vi "Untitled 5.vi"(8 "error in":errorcluster, 11 "Resources in":T1 {"ZI ModHandle"."ModHandle" format="0x%08x"; "ZI ModHandle"."Conn" format="0x%08x"; "ZI Handle"."Handle" format="0x%08x"; "ZI Handle"."Conn" format="0x%08x"}) -> (0 "error out":errorcluster, 2 "ZI Data":T4, 3 "Resources out":T1 {"ZI ModHandle"."ModHandle" format="0x%08x"; "ZI ModHandle"."Conn" format="0x%08x"; "ZI Handle"."Handle" format="0x%08x"; "ZI Handle"."Conn" format="0x%08x"})   [LabVIEW 2021]
uses:
  Main/Ver_1/ZI_Data.ctl
  Main/Ver_1/Resources.ctl
  <instrlib>/Zurich Instruments LabOne/Public/ziTypeHandle.ctl
  <instrlib>/Zurich Instruments LabOne/Public/Modules/ziTypeModHandle.ctl
  <instrlib>/Zurich Instruments LabOne/Public/Modules/ziModGetDoubleData.vi
  <instrlib>/Zurich Instruments LabOne/Public/Utility/ziTicksToS_vector.vi
  <instrlib>/Zurich Instruments LabOne/Zurich Instruments LabOne.lvlib
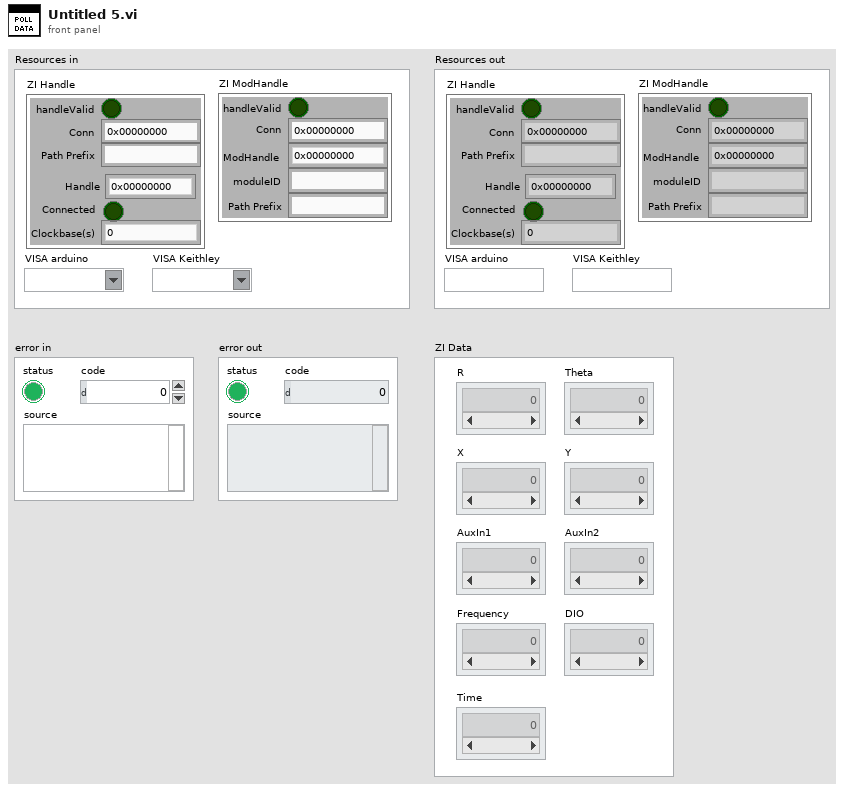
[diagram p1: front panel]
types:
  T1 = typedef "Resources.ctl" = cluster{"ZI Handle":T2, "ZI ModHandle":T3, "VISA arduino":refnum<visa-resource-name>, "VISA Keithley":refnum<visa-resource-name>}
  T2 = typedef "Zurich Instruments LabOne.lvlib/ziTypeHandle.ctl" = cluster{"handleValid":bool, "Conn":u64, "Path Prefix":string, "Handle":u64, "Connected":bool, "Clockbase(s)":dbl}
  T3 = typedef "Zurich Instruments LabOne.lvlib/ziTypeModHandle.ctl" = cluster{"handleValid":bool, "Conn":u64, "ModHandle":u64, "moduleID":string, "Path Prefix":string}
  T4 = typedef "ZI_Data.ctl" = cluster{"R":dbl[], "Theta":dbl[], "X":dbl[], "Y":dbl[], "AuxIn1":dbl[], "AuxIn2":dbl[], "Frequency":dbl[], "DIO":dbl[], "Time":dbl[]}
  T5 = typedef "Zurich Instruments LabOne.lvlib/ziTypeModResults.ctl" = cluster{"PathArray":string[], "ValueType":T6, "NoOfResults":u64, "ziGenericHeader":T7[]}
  T6 = typedef "Zurich Instruments LabOne.lvlib/ziTypePollType.ctl" = enum16{"NONE", "DOUBLE_DATA", "INTEGER_DATA", "DEMOD_SAMPLE", "SCOPE_WAVE_HF2", "AUXIN_SAMPLE", "DIO_SAMPLE", "BYTE_ARRAY", "PWA_WAVE", "9", "10", "11", "12", "13", "14", "15", "TREE_CHANGE_DEPRI", "17", "ERROR", "19", "20", "21", "22", "23", "24", "25", "26", "27", "28", "29", "30", "31", "DOUBLE_DATA_TS", "INTEGER_DATA_TS", "34", "SCOPE_WAVE", "SCOPE_WAVE_EX", "37", "BYTE_ARRAY_TS", "39", "40", "41", "42", "43", "44", "45", "CNT_DATA", "47", "TREE_CHANGE", "49", "50", "51", "52", "53", "54", "55", "56", "57", "58", "59", "60", "61", "62", "63", "SWEEPER_DATA", "SPECTRUM_DATA", "ADVISOR_DATA", "VECTOR_DATA", "IMP_DATA"}
  T7 = typedef "Zurich Instruments LabOne.lvlib/ziTypeModGenericHeader.ctl" = cluster{"HeaderType":enum8{"HEADER_TYPE_NONE", "HEADER_TYPE_SWTRIGGER", "HEADER_TYPE_SWEEPER"}, "SampleFormat":u8, "SystemTime":timestamp, "CreatedTimeStamp":u64, "ChangedTimeStamp":u64, "Flags":u32, "ChunkSizeBytes":u64, "Name":string, "Status":u32, "GroupIndex":u32, "Color":u32, "ActiveRow":u32, "TriggerNumber":u64, "GridRows":u32, "GridCols":u32, "GridMode":u32, "GridOperation":u32, "GridDirection":u32, "GridRepetitions":u32, "GridColDelta":dbl, "GridColOffset":dbl, "GridRowDelta":dbl, "GridRowOffset":dbl, "Bandwidth":dbl, "Center":dbl, "Nenbw":dbl}
  T8 = typedef "Zurich Instruments LabOne.lvlib/ziTypeDoubleDataTS.ctl" = cluster{"Timestamp (ticks)":u64[], "Value":dbl[]}
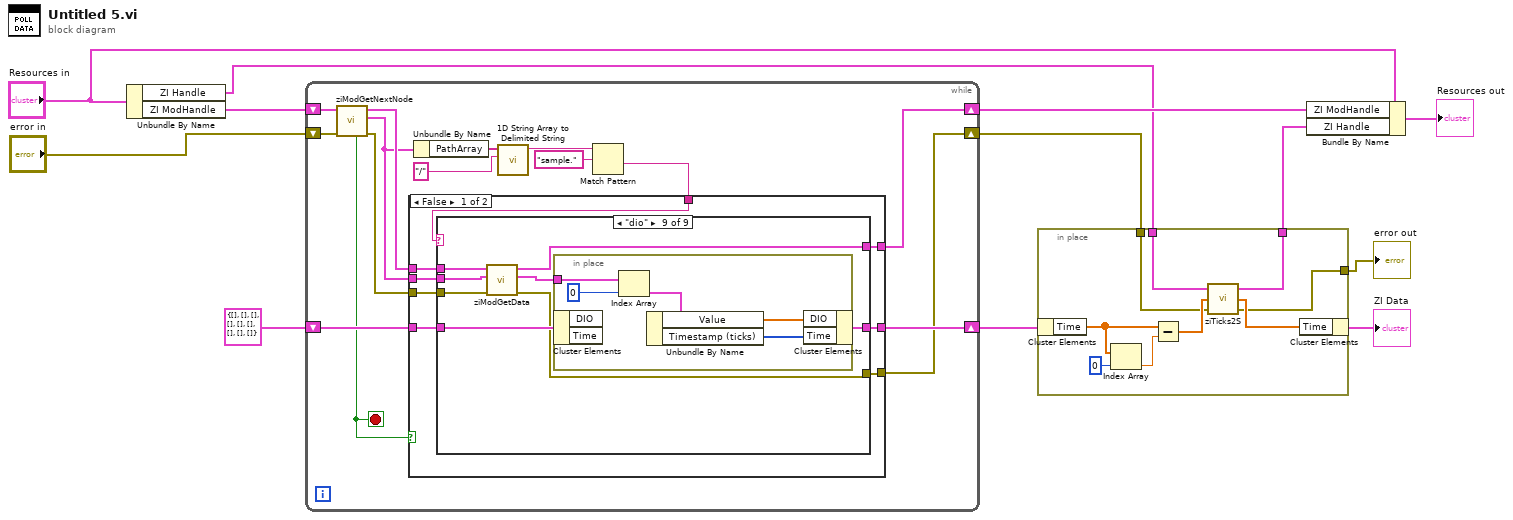
[diagram p0: block diagram]
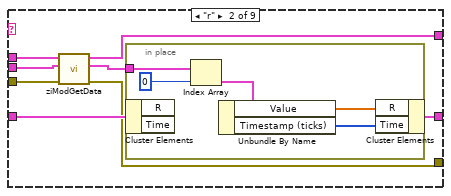
[diagram p3: hidden frame]
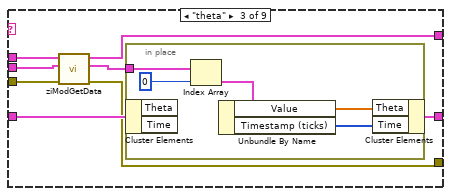
[diagram p4: hidden frame]
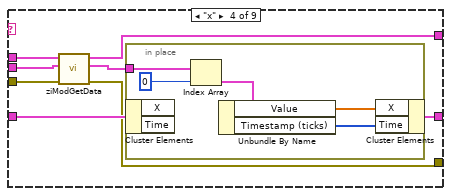
[diagram p5: hidden frame]
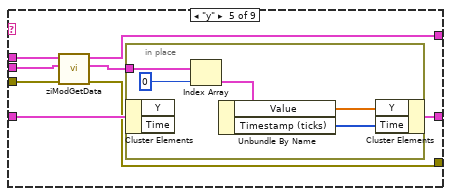
[diagram p6: hidden frame]
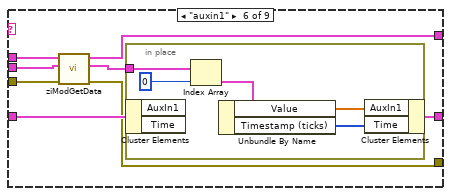
[diagram p7: hidden frame]
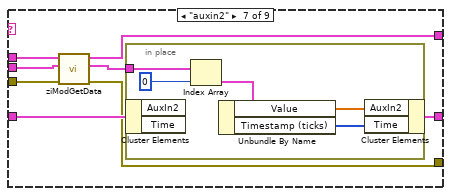
[diagram p8: hidden frame]
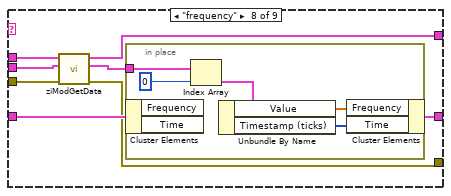
[diagram p9: hidden frame]
diagram:
  n1 = Unbundle By Name("Resources in") -> ("ZI Handle"=w8:T2, "ZI ModHandle"=w12:T3)
  n2 = while {
    shift-right: [w17] -> w10
    shift-left: w12 -> [w27]
    shift-right: [w16] -> w5
    shift-left: "error in" -> [w26]
    shift-right: [w18] -> w9
    shift-left: T4 {"R"=[], "Theta"=[], "X"=[], "Y"=[], "AuxIn1"=[], "AuxIn2"=[], "Frequency"=[], "DIO"=[], "Time"=[]} ("ZI Data") -> [w19]
    stop <- w15 stop-if-true
    n3 = call <instrlib>:"ziModGetNextNode.vi"("Error In"=w26, "ModHandle In"=w27) -> ("Error Out"=w22:errorcluster, "ModResults"=w20:T5, "ModHandle Out"=w21:T3, "NoData"=w15:bool)  [unwired: 6 in]
    n4 = Unbundle By Name(w20) -> ("PathArray"=w23:string[])
    n5 = call <vilib>:"1D String Array to Delimited String.vi"("delimiter"="/", "string array"=w23) -> ("delimited string"=w13:string)  [unwired: 9 in]
    n6 = Match Pattern(string=w13, regular expression="sample.") -> (after substring=w14:string)  [unwired: 1 in, 3 out]
    n7 = case shown="False" w15 {
      tunnel: w14 -> [w35 _]
      tunnel: w22 -> [w33 w144]
      tunnel: w21 -> [w34 w143]
      tunnel: w20 -> [w32 _]
      tunnel: w19 -> [w31 w145]
      tunnel: [w30 w145] -> w18
      tunnel: [w29 w143] -> w17
      tunnel: [w28 w144] -> w16
      frame False {
        n8 = case shown="\"dio\"" w35 {
          tunnel: w34 -> [w38 w46 w59 w72 w85 w98 w111 w124 w137]
          tunnel: w33 -> [w36 w45 w58 w71 w84 w97 w110 w123 w136]
          tunnel: w32 -> [_ w44 w57 w70 w83 w96 w109 w122 w135]
          tunnel: w31 -> [w37 w43 w56 w69 w82 w95 w108 w121 w134]
          tunnel: [w37 w41 w54 w67 w80 w93 w106 w119 w132] -> w30
          tunnel: [w38 w40 w53 w66 w79 w92 w105 w118 w131] -> w29
          tunnel: [w36 w39 w52 w65 w78 w91 w104 w117 w130] -> w28
          frame "", Default {
          }
          frame "r" {
            n9 = call-poly <instrlib>:"ziModGetData.vi"("Error In"=w45, "ModResults"=w44, "ModHandle In"=w46) -> ("Error Out"=w39:errorcluster, "DoubleSample"=w42:T8[], "ModHandle Out"=w40:T3)  [unwired: 4 in, 2 out]
            n10 = in-place {
              in-place-border: w42 -> [w51]
              n11 = in-place-cluster #1(w43) -> ()  [unwired: 2 out]
              n12 = Index Array(array=w51, index=0) -> (element=w49:T8)
              n13 = Unbundle By Name(w49) -> ("Value"=w48:dbl[], "Timestamp (ticks)"=w47:u64[])
              n14 = in-place-cluster #1("R"=w48, "Time"=w47) -> (w41:T4)
            }
          }
          frame "theta" {
            n15 = call-poly <instrlib>:"ziModGetData.vi"("Error In"=w58, "ModResults"=w57, "ModHandle In"=w59) -> ("Error Out"=w52:errorcluster, "DoubleSample"=w55:T8[], "ModHandle Out"=w53:T3)  [unwired: 4 in, 2 out]
            n16 = in-place {
              in-place-border: w55 -> [w64]
              n17 = in-place-cluster #2(w56) -> ()  [unwired: 2 out]
              n18 = Index Array(array=w64, index=0) -> (element=w62:T8)
              n19 = Unbundle By Name(w62) -> ("Value"=w61:dbl[], "Timestamp (ticks)"=w60:u64[])
              n20 = in-place-cluster #2("Theta"=w61, "Time"=w60) -> (w54:T4)
            }
          }
          frame "x" {
            n21 = call-poly <instrlib>:"ziModGetData.vi"("Error In"=w71, "ModResults"=w70, "ModHandle In"=w72) -> ("Error Out"=w65:errorcluster, "DoubleSample"=w68:T8[], "ModHandle Out"=w66:T3)  [unwired: 4 in, 2 out]
            n22 = in-place {
              in-place-border: w68 -> [w77]
              n23 = in-place-cluster #3(w69) -> ()  [unwired: 2 out]
              n24 = Index Array(array=w77, index=0) -> (element=w75:T8)
              n25 = Unbundle By Name(w75) -> ("Value"=w74:dbl[], "Timestamp (ticks)"=w73:u64[])
              n26 = in-place-cluster #3("X"=w74, "Time"=w73) -> (w67:T4)
            }
          }
          frame "y" {
            n27 = call-poly <instrlib>:"ziModGetData.vi"("Error In"=w84, "ModResults"=w83, "ModHandle In"=w85) -> ("Error Out"=w78:errorcluster, "DoubleSample"=w81:T8[], "ModHandle Out"=w79:T3)  [unwired: 4 in, 2 out]
            n28 = in-place {
              in-place-border: w81 -> [w90]
              n29 = in-place-cluster #4(w82) -> ()  [unwired: 2 out]
              n30 = Index Array(array=w90, index=0) -> (element=w88:T8)
              n31 = Unbundle By Name(w88) -> ("Value"=w87:dbl[], "Timestamp (ticks)"=w86:u64[])
              n32 = in-place-cluster #4("Y"=w87, "Time"=w86) -> (w80:T4)
            }
          }
          frame "auxin1" {
            n33 = call-poly <instrlib>:"ziModGetData.vi"("Error In"=w97, "ModResults"=w96, "ModHandle In"=w98) -> ("Error Out"=w91:errorcluster, "DoubleSample"=w94:T8[], "ModHandle Out"=w92:T3)  [unwired: 4 in, 2 out]
            n34 = in-place {
              in-place-border: w94 -> [w103]
              n35 = in-place-cluster #5(w95) -> ()  [unwired: 2 out]
              n36 = Index Array(array=w103, index=0) -> (element=w101:T8)
              n37 = Unbundle By Name(w101) -> ("Value"=w100:dbl[], "Timestamp (ticks)"=w99:u64[])
              n38 = in-place-cluster #5("AuxIn1"=w100, "Time"=w99) -> (w93:T4)
            }
          }
          frame "auxin2" {
            n39 = call-poly <instrlib>:"ziModGetData.vi"("Error In"=w110, "ModResults"=w109, "ModHandle In"=w111) -> ("Error Out"=w104:errorcluster, "DoubleSample"=w107:T8[], "ModHandle Out"=w105:T3)  [unwired: 4 in, 2 out]
            n40 = in-place {
              in-place-border: w107 -> [w116]
              n41 = in-place-cluster #6(w108) -> ()  [unwired: 2 out]
              n42 = Index Array(array=w116, index=0) -> (element=w114:T8)
              n43 = Unbundle By Name(w114) -> ("Value"=w113:dbl[], "Timestamp (ticks)"=w112:u64[])
              n44 = in-place-cluster #6("AuxIn2"=w113, "Time"=w112) -> (w106:T4)
            }
          }
          frame "frequency" {
            n45 = call-poly <instrlib>:"ziModGetData.vi"("Error In"=w123, "ModResults"=w122, "ModHandle In"=w124) -> ("Error Out"=w117:errorcluster, "DoubleSample"=w120:T8[], "ModHandle Out"=w118:T3)  [unwired: 4 in, 2 out]
            n46 = in-place {
              in-place-border: w120 -> [w129]
              n47 = in-place-cluster #7(w121) -> ()  [unwired: 2 out]
              n48 = Index Array(array=w129, index=0) -> (element=w127:T8)
              n49 = Unbundle By Name(w127) -> ("Value"=w126:dbl[], "Timestamp (ticks)"=w125:u64[])
              n50 = in-place-cluster #7("Frequency"=w126, "Time"=w125) -> (w119:T4)
            }
          }
          frame "dio" {
            n51 = call-poly <instrlib>:"ziModGetData.vi"("Error In"=w136, "ModResults"=w135, "ModHandle In"=w137) -> ("Error Out"=w130:errorcluster, "DoubleSample"=w133:T8[], "ModHandle Out"=w131:T3)  [unwired: 4 in, 2 out]
            n52 = in-place {
              in-place-border: w133 -> [w142]
              n53 = in-place-cluster #8(w134) -> ()  [unwired: 2 out]
              n54 = Index Array(array=w142, index=0) -> (element=w140:T8)
              n55 = Unbundle By Name(w140) -> ("Value"=w139:dbl[], "Timestamp (ticks)"=w138:u64[])
              n56 = in-place-cluster #8("DIO"=w139, "Time"=w138) -> (w132:T4)
            }
          }
        }
      }
      frame True {
      }
    }
  }
  n57 = in-place {
    in-place-border: w8 -> [w151]
    in-place-border: [w148] -> w7
    in-place-border: w5 -> [w147]
    in-place-border: [w146] -> w1
    n58 = in-place-cluster #9(w9) -> ("Time"=w152:dbl[])
    n59 = Index Array(array=w152, index=0) -> (element=w153:dbl)
    n60 = Subtract(x=w152, y=w153) -> (x-y=w150:dbl[])
    n61 = call-poly <instrlib>:"ziTicks2S.vi"("Error In"=w147, "Timestamp (ticks)"=w150, "Handle In"=w151) -> ("Error Out"=w146:errorcluster, "Timestamp(s)"=w149:dbl[], "Handle Out"=w148:T2)
    n62 = in-place-cluster #9("Time"=w149) -> (→"ZI Data":T4)
  }
  "error out" <- w1
  n63 = Bundle By Name(cluster="Resources in", "ZI ModHandle"=w10, "ZI Handle"=w7) -> (→"Resources out":T1)
